vi "EXE1.vi"() -> ()   [LabVIEW 2016]
uses:
  <vilib>/measure/mamon.llb/Create Continuous Mask using Formula.vi
  <vilib>/xnet/xnet.llb/XNET Read (Signal Waveform) .vi
  <vilib>/measure/mamon.llb/Limit Testing Time.vi
  <vilib>/xnet/xnet.llb/XNET Write (Signal Single-point).vi
  <vilib>/xnet/xnet.llb/XNET Read (Signal Single-point).vi
  <vilib>/measure/NI_MAPro.lvlib
  <vilib>/measure/NI_MABase.lvlib
  <vilib>/measure/mamon.llb/Create Continuous Mask.vi
panel:
  out "data":dbl[](array[numeric]) format="%.2f"
  in  "frequency":dbl=10.0 format="%0.2p"
  in  "signal type":T1(ring)
  out "Waveform Chart":dbl(graph)
  out "Waveform Chart 2":waveform(dbl)[](graph)
  out "Boolean":bool
  in  "Data":dbl[](array[numeric])=[0.0]
  in  "Menu":dbl[](array[numeric])=[0.0]
  in  "Fuction":dbl[](array[numeric])=[0.0]
  in  "Frequency":dbl[](array[numeric])=[0.0]
  in  "Contrast":dbl[](array[numeric])=[0.0]
  in  "milliseconds to wait":u32=100
  in  "stop":bool
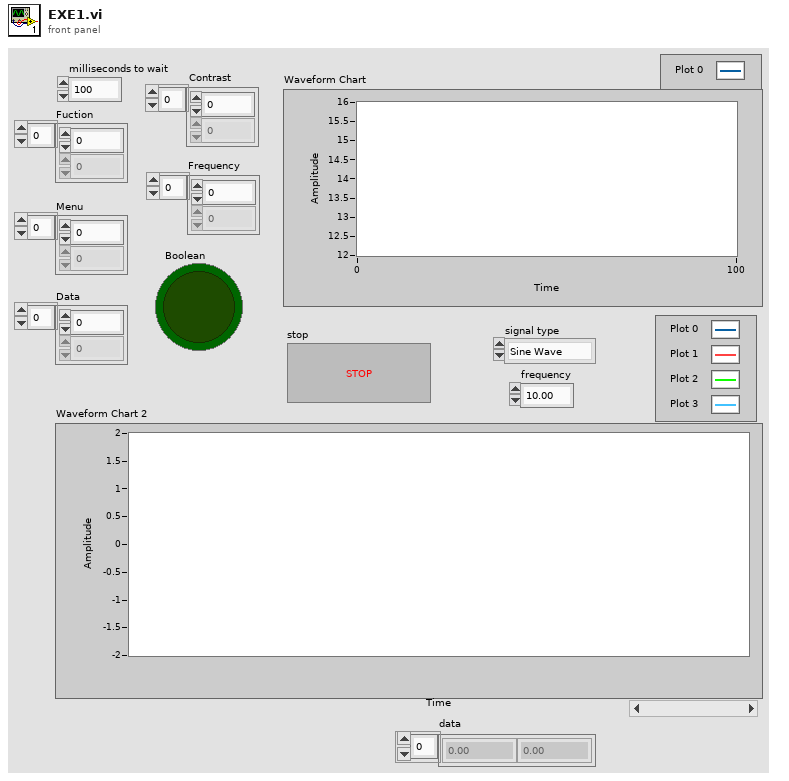
[diagram p1: front panel]
types:
  T1 = enum16{"Sine Wave", "Triangle Wave", "Square Wave", "Sawtooth Wave"}
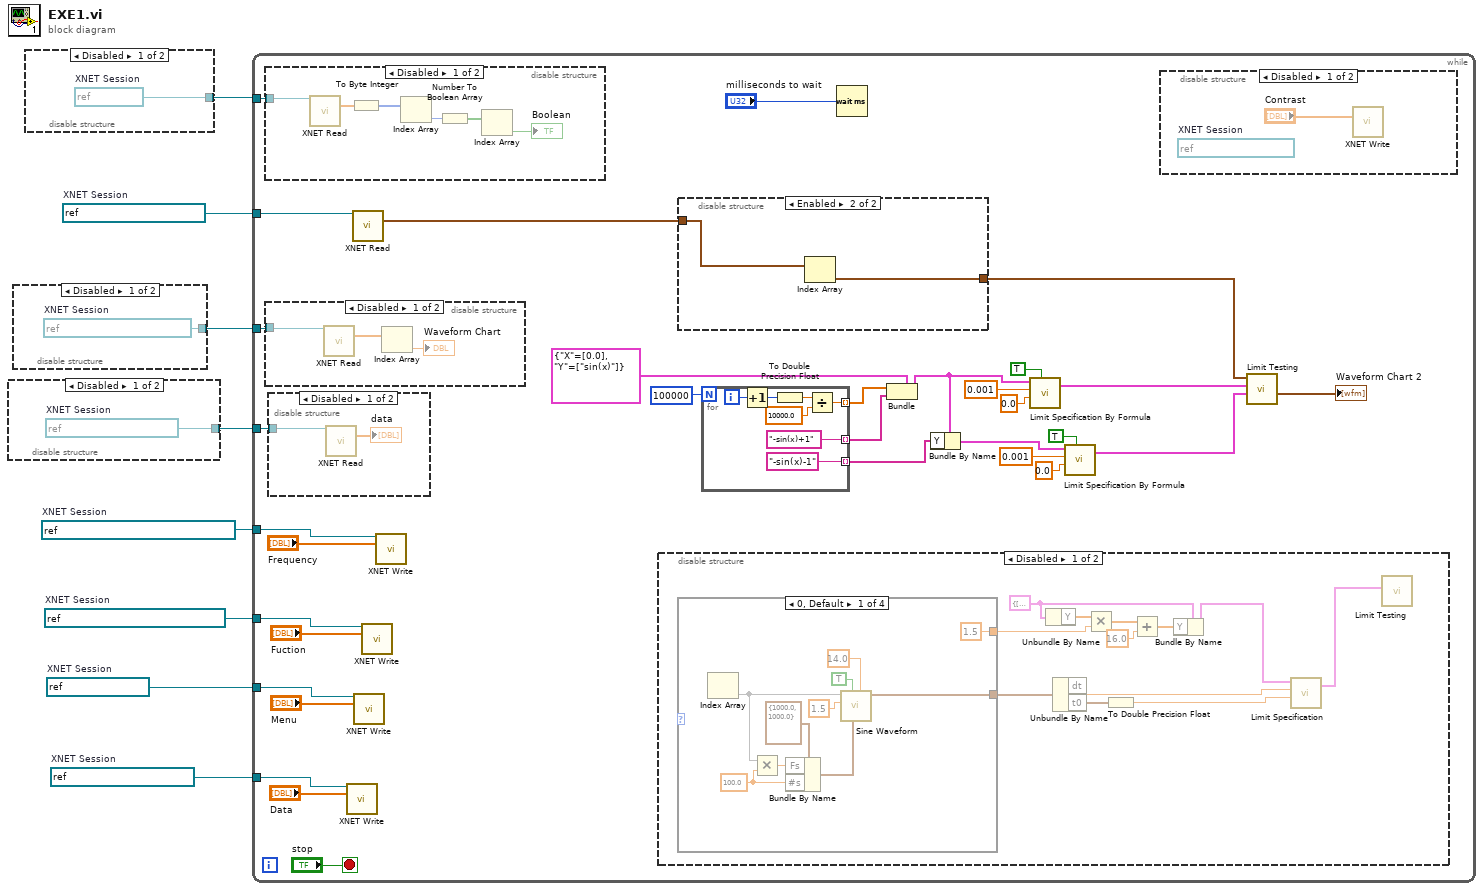
[diagram p0: block diagram]
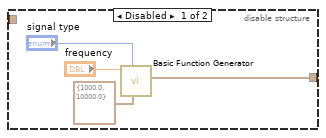
[diagram p7: hidden frame]
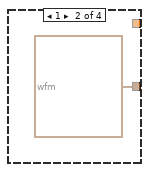
[diagram p9: hidden frame]
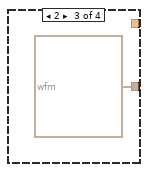
[diagram p10: hidden frame]
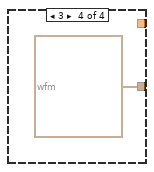
[diagram p11: hidden frame]
diagram:
  w1 = refnum<k21> "New NI-XNET Session"  # XNET Session
  w4 = refnum<k21> "String Request to CDB"  # XNET Session
  w5 = refnum<k21> "Set LCD Menu"  # XNET Session
  w6 = refnum<k21> "Function Generation Selector"  # XNET Session
  w7 = refnum<k21> "Function Generation Frequency"  # XNET Session
  n1 = disable-structure shown="Disabled" {
    disable-tunnel: [w9 _] -> w2
    frame Disabled {
      w9 = refnum<k21> "Function Frequency"  # XNET Session
    }
    frame Enabled {
    }
  }
  n2 = disable-structure shown="Disabled" {
    disable-tunnel: [w10 _] -> w3
    frame Disabled {
      w10 = refnum<k21> "Analog In To CAN Ch1"  # XNET Session
    }
    frame Enabled {
    }
  }
  n3 = disable-structure shown="Disabled" {
    disable-tunnel: [w11 _] -> w8
    frame Disabled {
      w11 = refnum<k21> "Switch0"  # XNET Session
    }
    frame Enabled {
    }
  }
  n4 = while {
    tunnel: w8 -> [w43]
    tunnel: w7 -> [w40]
    tunnel: w6 -> [w39]
    tunnel: w5 -> [w37]
    tunnel: w4 -> [w35]
    tunnel: w3 -> [w34]
    tunnel: w2 -> [w15]
    tunnel: w1 -> [w14]
    stop <- "stop" stop-if-true
    n5 = disable-structure shown="Disabled" {
      disable-tunnel: w43 -> [w60 _]
      frame Disabled {
        n6 = call-poly <vilib>:"XNET Read.vi"("session in"=w60) -> ("data"=w57:dbl[])  [unwired: 12 in, 2 out]
        n7 = To Byte Integer(number=w57) -> (8bit integer=w56:i8[])
        n8 = Index Array(array=w56) -> (element=w55:i8)  [unwired: 1 in]
        n9 = Number To Boolean Array(number=w55) -> (Boolean array=w59:bool[])
        n10 = Index Array(array=w59) -> (element=→"Boolean":bool)  [unwired: 1 in]
      }
      frame Enabled {
      }
    }
    n11 = disable-structure shown="Disabled" {
      disable-tunnel: w34 -> [w48 _]
      frame Disabled {
        n12 = call-poly <vilib>:"XNET Read.vi"("session in"=w48) -> ("data"=w47:dbl[])  [unwired: 12 in, 2 out]
        n13 = Index Array(array=w47) -> (element=→"Waveform Chart":dbl)  [unwired: 1 in]
      }
      frame Enabled {
      }
    }
    n14 = disable-structure shown="Disabled" {
      disable-tunnel: w15 -> [w45 _]
      frame Disabled {
        n15 = call-poly <vilib>:"XNET Read.vi"("session in"=w45) -> ("data"=→"data":dbl[])  [unwired: 12 in, 2 out]
      }
      frame Enabled {
      }
    }
    n16 = call-poly <vilib>:"XNET Write.vi"("session in"=w35, "data"="Data") -> ()  [unwired: 12 in, 2 out]
    n17 = call-poly <vilib>:"XNET Read.vi"("session in"=w14) -> ("data"=w12:waveform(dbl)[])  [unwired: 12 in, 2 out]
    n18 = call-poly <vilib>:"XNET Write.vi"("session in"=w37, "data"="Menu") -> ()  [unwired: 12 in, 2 out]
    n19 = call-poly <vilib>:"XNET Write.vi"("session in"=w39, "data"="Fuction") -> ()  [unwired: 12 in, 2 out]
    n20 = call-poly <vilib>:"XNET Write.vi"("session in"=w40, "data"="Frequency") -> ()  [unwired: 12 in, 2 out]
    n21 = disable-structure shown="Disabled" {
      frame Disabled {
        w75 = cluster{"X":dbl[], "Y":dbl[]} {"X"=[0.0, 1.0, 2.0, 3.0, 4.0, 5.0, 6.0, 7.0, 8.0, 9.0, 10.0, 11.0, 12.0, 13.0, 14.0, 15.0, 16.0, 17.0, 18.0, 19.0, 20.0, 21.0, 22.0, 23.0, 24.0, 25.0, 26.0, 27.0, 28.0, 29.0, 30.0, 31.0, 32.0, 33.0, 34.0, 35.0, 36.0, 37.0, 38.0, 39.0, 40.0, 41.0, 42.0, 43.0, 44.0, 45.0, 46.0, 47.0, 48.0, 49.0, 50.0, 51.0, 52.0, 53.0, 54.0, 55.0, 56.0, 57.0, 58.0, 59.0, 60.0, 61.0, 62.0, 63.0, 64.0, 65.0, 66.0, 67.0, 68.0, 69.0, 70.0, 71.0, 72.0, 73.0, 74.0, 75.0, 76.0, 77.0, 78.0, 79.0, 80.0, 81.0, 82.0, 83.0, 84.0, 85.0, 86.0, 87.0, 88.0, 89.0, 90.0, 91.0, 92.0, 93.0, 94.0, 95.0, 96.0, 97.0, 98.0, 99.0], "Y"=[0.0, 0.06279051952931337, 0.12533323356430423, 0.18738131458572463, 0.2486898871648548, 0.30901699437494745, 0.368124552684678, 0.42577929156507266, 0.4817536741017153, 0.5358267949789967, 0.5877852522924731, 0.6374239897486897, 0.6845471059286887, 0.7289686274214116, 0.7705132427757893, 0.8090169943749475, 0.8443279255020151, 0.8763066800438636, 0.9048270524660196, 0.9297764858882515, 0.9510565162951536, 0.9685831611286312, 0.9822872507286887, 0.9921147013144779, 0.9980267284282716, 1.0, 0.9980267284282716, 0.9921147013144779, 0.9822872507286887, 0.9685831611286312, 0.9510565162951536, 0.9297764858882515, 0.9048270524660196, 0.8763066800438637, 0.8443279255020151, 0.8090169943749476, 0.7705132427757893, 0.7289686274214117, 0.6845471059286887, 0.6374239897486899, 0.5877852522924731, 0.5358267949789968, 0.48175367410171527, 0.4257792915650728, 0.3681245526846779, 0.3090169943749476, 0.24868988716485474, 0.18738131458572485, 0.1253332335643042, 0.06279051952931362, -2.7755575615628914e-17, -0.0627905195293131, -0.12533323356430426, -0.18738131458572432, -0.2486898871648548, -0.3090169943749471, -0.368124552684678, -0.4257792915650723, -0.4817536741017153, -0.5358267949789963, -0.5877852522924731, -0.6374239897486894, -0.6845471059286887, -0.7289686274214112, -0.7705132427757893, -0.8090169943749471, -0.8443279255020151, -0.8763066800438633, -0.9048270524660196, -0.9297764858882511, -0.9510565162951536, -0.9685831611286309, -0.9822872507286887, -0.9921147013144775, -0.9980267284282716, -0.9999999999999998, -0.9980267284282716, -0.9921147013144777, -0.9822872507286887, -0.968583161128631, -0.9510565162951536, -0.9297764858882513, -0.9048270524660196, -0.8763066800438636, -0.8443279255020151, -0.8090169943749475, -0.7705132427757893, -0.7289686274214116, -0.6845471059286887, -0.6374239897486897, -0.5877852522924731, -0.5358267949789967, -0.48175367410171527, -0.4257792915650727, -0.3681245526846779, -0.30901699437494756, -0.24868988716485474, -0.18738131458572482, -0.1253332335643042, -0.06279051952931361]} ("output cluster 2")
        n22 = case shown="0, Default" {
          selector: _ -> [_ _ _ _]
          tunnel: [w83 waveform(dbl) {"t0"=timestamp(0 s since 1904-01-01), "dt"=1.0, "Y"=[]} ("signal out") waveform(dbl) {"t0"=timestamp(0 s since 1904-01-01), "dt"=1.0, "Y"=[]} ("signal out") waveform(dbl) {"t0"=timestamp(0 s since 1904-01-01), "dt"=1.0, "Y"=[]} ("signal out")] -> w79
          tunnel: [1.5 ("amplitude") _ _ _] -> w72
          frame 0, Default {
            w89 = 100.0 ("y")
            n23 = Index Array() -> (element=w85)  [unwired: 2 in]
            n24 = Multiply(x=w85, y=w89) -> (x*y=w88:dbl)
            n25 = Bundle By Name(cluster=cluster{"Fs":dbl, "#s":dbl} {"Fs"=1000.0, "#s"=1000.0} ("sampling info"), "Fs"=w88, "#s"=w89) -> (w87:cluster{"Fs":dbl, "#s":dbl})
            n26 = call <vilib>:"Sine Waveform.vi"("offset"=14.0, "sampling info"=w87, "reset signal"=TRUE, "amplitude"=1.5, "frequency"=w85) -> ("signal out"=w83:waveform(dbl))  [unwired: 5 in, 1 out]
          }
          frame 1 {
          }
          frame 2 {
          }
          frame 3 {
          }
        }
        n27 = Unbundle By Name(w75) -> ("Y"=w73:dbl[])
        n28 = Unbundle By Name(w79) -> ("dt"=w78:dbl, "t0"=w77:timestamp)
        n29 = Multiply(x=w73, y=w72) -> (x*y=w70:dbl[])
        n30 = To Double Precision Float(number=w77) -> (double precision float=w76:dbl)
        n31 = Add(x=w70, y=16.0 ("offset")) -> (x+y=w71:dbl[])
        n32 = Bundle By Name(cluster=w75, "Y"=w71) -> (w74:cluster{"X":dbl[], "Y":dbl[]})
        n33 = call-poly <vilib>:"Limit Specification.vi"("Specification Cluster"=w74, "dx"=w78, "x0"=w76) -> ("Limit"=w68:cluster{"x0":dbl, "dx":dbl, "Y":dbl[]})  [unwired: 2 in, 1 out]
        n34 = call-poly <vilib>:"Limit Testing.vi"("upper limit"=w68) -> ()  [unwired: 5 in, 6 out]
      }
      frame Enabled {
      }
    }
    n35 = disable-structure shown="Enabled" {
      disable-tunnel: [w51 w53] -> w13
      disable-tunnel: w12 -> [_ w54]
      frame Disabled {
        n36 = call <vilib>:"Basic Function Generator.vi"("sampling info"=cluster{"Fs":dbl, "#s":dbl} {"Fs"=1000.0, "#s"=10000.0}, "signal type"="signal type", "frequency"="frequency") -> ("signal out"=w51:waveform(dbl))  [unwired: 6 in, 2 out]
      }
      frame Enabled {
        n37 = Index Array(array=w54) -> (element=w53:waveform(dbl))  [unwired: 1 in]
      }
    }
    n38 = for {
      N: 100000 -> [_]
      tunnel: [w67] -> w23 mode=indexing
      tunnel: ["-sin(x)+1" ("String")] -> w25 mode=indexing
      tunnel: ["-sin(x)-1" ("String")] -> w32 mode=indexing
      i -> [w64]
      n39 = Increment(x=w64) -> (x+1=w66:i32)
      n40 = To Double Precision Float(number=w66) -> (double precision float=w63:dbl)
      n41 = Divide(x=w63, y=10000.0) -> (x/y=w67:dbl)
    }
    n42 = Wait (ms)(milliseconds to wait="milliseconds to wait") -> ()  [unwired: 1 out]
    n43 = Bundle(cluster=cluster{"X":dbl[], "Y":string[]} {"X"=[0.0], "Y"=["sin(x)"]} ("Specification Cluster"), "X"=w23, "Y"=w25) -> (w30:cluster{"X":dbl[], "Y":string[]})
    n44 = Bundle By Name(cluster=w30, "Y"=w32) -> (w31:cluster{"X":dbl[], "Y":string[]})
    n45 = call-poly <vilib>:"Limit Specification By Formula.vi"("Specification Cluster"=w30, "dx"=0.001, "x0"=0.0, "Reset"=TRUE) -> ("Limit"=w26:cluster{"x0":dbl, "dx":dbl, "Y":dbl[]})  [unwired: 1 in, 1 out]
    n46 = call-poly <vilib>:"Limit Specification By Formula.vi"("Specification Cluster"=w31, "dx"=0.001, "x0"=0.0, "Reset"=TRUE) -> ("Limit"=w29:cluster{"x0":dbl, "dx":dbl, "Y":dbl[]})  [unwired: 1 in, 1 out]
    n47 = disable-structure shown="Disabled" {
      frame Disabled {
        (unwired) refnum<k21> "Set LCD Contrast"  # XNET Session
        n48 = call-poly <vilib>:"XNET Write.vi"("data"="Contrast") -> ()  [unwired: 13 in, 2 out]
      }
      frame Enabled {
      }
    }
    n49 = call-poly <vilib>:"Limit Testing.vi"("lower limit"=w29, "upper limit"=w26, "signal in"=w13) -> ("output values"=→"Waveform Chart 2":waveform(dbl)[])  [unwired: 3 in, 5 out]
  }
